vi "Harvester Intake.vi"(3 "Joy Val":dbl) -> ()   [LabVIEW 2015]
panel:
  in  "Harvester Out":dbl(slide)=1.0 scale=0.0..1.0
  in  "Harvester In":dbl(slide)=1.0 scale=0.0..1.0
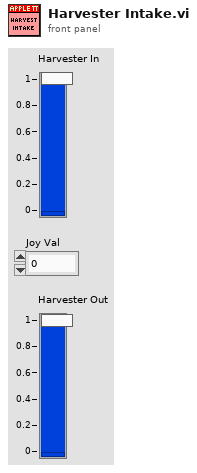
[diagram p1: front panel]
types:
  T1 = typedef "WPI_MotorControlDeviceRef.ctl" = cluster{"DeviceStatus":errorcluster, "Type":T2, "PWM":cluster{"PWM Channel":T3, "DeadBand":T4}, "CAN":cluster{"Device Number":u8, "Control Mode":T5, "Semaphore":T6, "Max Vout":dbl, "TalonSRX Control Mode":T7}, "Invert":bool}
  T2 = typedef "WPI_MotorControlType.ctl" = enum16{"PWM", "CAN", "CANTalonSRX"}
  T3 = typedef "FPGA_DIOPWMChannel.ctl" = enum8{"PWM 0", "PWM 1", "PWM 2", "PWM 3", "PWM 4", "PWM 5", "PWM 6", "PWM 7", "PWM 8", "PWM 9", "PWM MXP 0", "PWM MXP 1", "PWM MXP 2", "PWM MXP 3", "PWM MXP 4", "PWM MXP 5", "PWM MXP 6", "PWM MXP 7", "PWM MXP 8", "PWM MXP 9", "Invalid"}
  T4 = typedef "WPI_PWMDeadband.ctl" = cluster{"Name":string, "maxPositivePwm":i32, "minPositivePwm":i32, "centerPwm":i32, "maxNegativePwm":i32, "minNegativePwm":i32, "angularRange":u16}
  T5 = typedef "WPI_CANJaguar_ControlMode.ctl" = enum8{"Percent VBus", "Current", "Speed", "Position", "Voltage"}
  T6 = typedef "Semaphore RefNum" = refnum<k1>
  T7 = typedef "WPI_CANTalonSRX_APIControlMode.ctl" = enum8{"Percent VBus", "Speed", "Position", "Slave", "Unchanged / Invalid", "Voltage Compensation", "Current", "Motion Profile"}
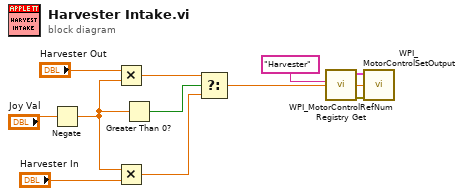
[diagram p0: block diagram]
diagram:
  n1 = Negate(x="Joy Val") -> (-x=w1:dbl)
  n2 = Multiply(x="Harvester Out", y=w1) -> (x*y=w9:dbl)
  n3 = Multiply(x=w1, y="Harvester In") -> (x*y=w7:dbl)
  n4 = Greater Than 0?(x=w1) -> (x > 0?=w6:bool)
  n5 = Select(t=w9, s=w6, f=w7) -> (s? t:f=w10:dbl)
  n6 = call <vilib>:"WPI_MotorControlRefNum Registry Get.vi"("refnum name"="Harvester") -> ("error out"=w4:errorcluster, "MotorControlDevRef"=w3:T1)  [unwired: 9 in]
  n7 = call <vilib>:"WPI_MotorControlSetOutput.vi"("error in (no error)"=w4, "Output"=w10, "MotorControlDevRef"=w3) -> ()  [unwired: 6 in, 3 out]
